vi "Refresh Info.vi"(8 "error in (no error)":errorcluster, 11 "Stepper3D in":refnum<class "Stepper3D.lvclass">) -> (0 "error out":errorcluster, 2 "status":T1, 3 "Stepper3D out":refnum<class "Stepper3D.lvclass">)   [LabVIEW 2014, in "Stepper3D.lvclass"]
uses:
  Stepper3D.lvclass
  Libs/stepper3D.lib/Enums/CurrentStatus.ctl
  Libs/stepper3D.lib/Enums/BoundaryStatus.ctl
  Stepper3D.lvclass/Stepper3D.ctl
  Framework/Interfaces/Observable Actor/Observable Actor.lvclass
  Libs/stepper3D.lib/stepper3D.lvlib
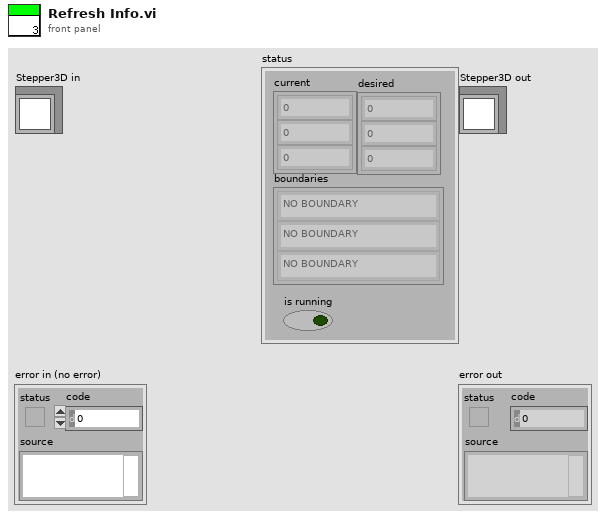
[diagram p1: front panel]
types:
  T1 = typedef "stepper3D.lvlib/CurrentStatus.ctl" = cluster{"desired":dbl[], "current":dbl[], "boundaries":T2[], "is running":bool}
  T2 = typedef "stepper3D.lvlib/BoundaryStatus.ctl" = enum16{"NO BOUNDARY", "OUT OF LEFT", "OUT OF RIGHT"}
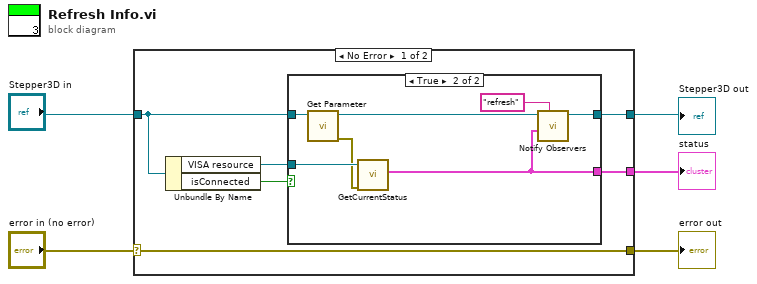
[diagram p0: block diagram]
diagram:
  n1 = case shown="No Error" "error in (no error)" {
    selector: "error in (no error)" -> [w11 w21]
    tunnel: [w11 w21] -> w4
    tunnel: [w7 w20] -> w2
    tunnel: "Stepper3D in" -> [w8 w20]
    tunnel: [w6 _] -> w1
    frame No Error {
      n2 = Unbundle By Name(w8) -> ("VISA resource"=w10:refnum<visa-resource-name>, "isConnected"=w9:bool)
      n3 = case shown="True" w9 {
        tunnel: w10 -> [_ w16]
        tunnel: w8 -> [w12 w18]
        tunnel: [w12 w13] -> w7
        tunnel: [_ w14] -> w6
        frame False {
        }
        frame True {
          n4 = call-dynamic "Get Parameter.vi"("Stepper3D in"=w18) -> ("error out"=w15:errorcluster, "Stepper3D out"=w17:refnum<class "Stepper3D.lvclass">)  [unwired: 8 in, 1 out]
          n5 = call "GetCurrentStatus.vi"("error in (no error)"=w15, "VISA Refnum in"=w16) -> ("status"=w14:T1)  [unwired: 7 in, 2 out]
          n6 = call "Notify Observers.vi"("name"="refresh", "value"=w14, "Observable Actor in"=w17) -> ("Observable Actor out"=w13:refnum<class "Stepper3D.lvclass">)  [unwired: 7 in, 1 out]
        }
      }
    }
    frame Error {
    }
  }
  "error out" <- w4
  "Stepper3D out" <- w2
  "status" <- w1
